vi "Reset Actuator.vi"(8 "error in":errorcluster, 9 "Time to wait":i32=999, 10 "Actuator Name":string, 11 "UTP IO Session in":T1) -> (0 "error out":errorcluster, 2 "ExpiredTimeToWait?":bool, 3 "UTP IO Session out":T1)   [LabVIEW 2023, in "Actuators.lvlib"]
doc: "Reset Actuator"
uses:
  Actuators.lvlib
  <vilib>/Noffz/UTP IO/UTP IO Library/Typedefs/Session Handle.ctl
  <vilib>/Noffz/UTP IO/UTP IO Library/UTP IO Pool Session.lvclass
  <vilib>/Noffz/UTP IO/UTP IO Library/methods/poly/plc/Write PLC Variable (Boolean).vi
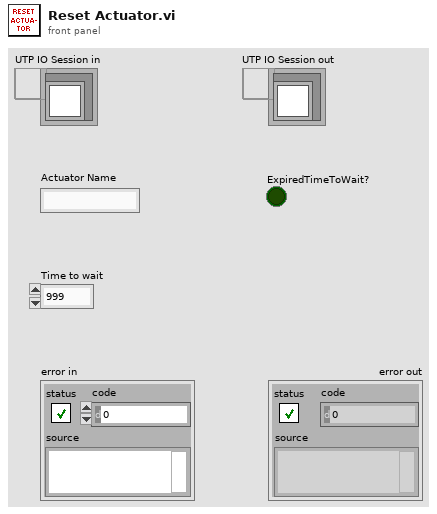
[diagram p1: front panel]
types:
  T1 = typedef "UTP IO Library.lvlib/UTP IO Pool Session.lvclass/Session Handle.ctl" = refnum<data-value>
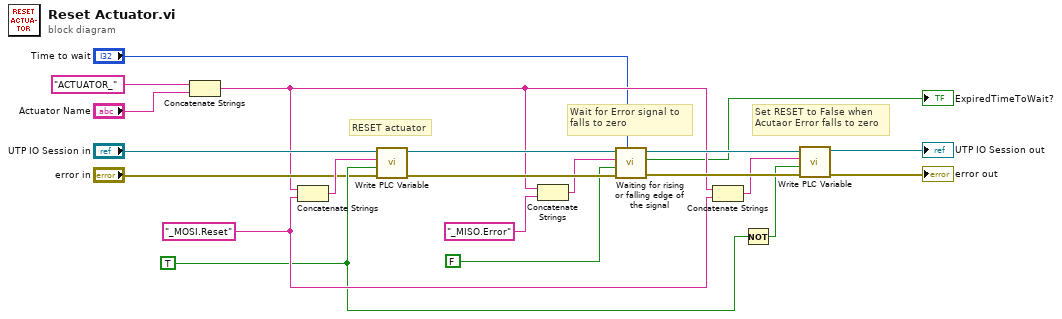
[diagram p0: block diagram]
diagram:
  w12 = TRUE ("value")
  w15 = "_MOSI.Reset" ("string")
  # "Set RESET to False when\nAcutaor Error falls to zero"
  # "Wait for Error signal to \nfalls to zero"
  # "RESET actuator"
  n1 = Concatenate Strings("ACTUATOR_" ("string"), "Actuator Name") -> (w5:string)
  n2 = Concatenate Strings(w5, w15) -> (w21:string)
  n3 = call-poly <vilib>:"Write PLC Variable.vi"("error in (no error)"="error in", "value"=w12, "variable name"=w21, "UTP IO Session in"="UTP IO Session in") -> ("error out"=w19:errorcluster, "UTP IO Session out"=w20:T1)  [unwired: 6 in]
  n4 = Concatenate Strings(w5, "_MISO.Error" ("string")) -> (w10:string)
  n5 = call "Waiting for rising or falling edge of the signal.vi"("Time to wait"="Time to wait", "error in"=w19, "Rising/Falling edge"=FALSE, "Variable name"=w10, "UTP IO Session in"=w20) -> ("error out"=w16:errorcluster, "ExpiredTimeToWait?"=→"ExpiredTimeToWait?":bool, "UTP IO Session out"=w17:T1)  [unwired: 4 in]
  n6 = Concatenate Strings(w5, w15) -> (w14:string)
  n7 = Not(x=w12) -> (.not. x?=w13:bool)
  n8 = call-poly <vilib>:"Write PLC Variable.vi"("error in (no error)"=w16, "value"=w13, "variable name"=w14, "UTP IO Session in"=w17) -> ("error out"=→"error out":errorcluster, "UTP IO Session out"=→"UTP IO Session out":T1)  [unwired: 6 in]
